vi "Bind RPC Register.vi"(11 "gRPCid server in":T1) -> (0 "error out":errorcluster, 1 "Register Internal UE":refnum<user-event>, 2 "Register gRPC UE":refnum<user-event>, 3 "gRPCid server out":T1)   [LabVIEW 2019, in "OOP Server.lvclass"]
uses:
  OOP Server.lvclass
  gRPC interface/Server API/typeDefs/gRPCId Cluster.ctl
  gRPC interface/Server API/typeDefs/grpcId.ctl
  typeDefs/gRPC Server Internal Message.ctl
  616620f9-6bbe-466a-af51-04bcc3596ea0.vi
  gRPC interface/gprc-lvsupport.lvlib
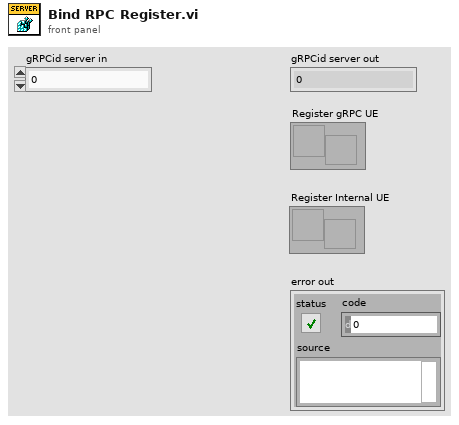
[diagram p1: front panel]
types:
  T1 = typedef "gprc-lvsupport.lvlib/grpcId.ctl" = u64
  T2 = typedef "OOP Server.lvclass/gRPC Server Internal Message.ctl" = cluster{"Command":string, "Data":variant}
  T3 = typedef "gprc-lvsupport.lvlib/gRPCId Cluster.ctl" = cluster{"gRPCid":T1}
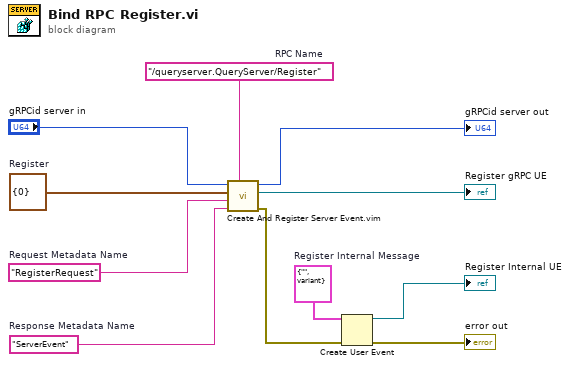
[diagram p0: block diagram]
diagram:
  w4 = T2 {"Command"="", "Data"=variant}  # Register Internal Message
  w7 = "ServerEvent"  # Response Metadata Name
  w10 = T3 {"gRPCid"=0}  # Register
  w8 = "RegisterRequest"  # Request Metadata Name
  w9 = "/queryserver.QueryServer/Register"  # RPC Name
  n1 = call "Create And Register Server Event.vim"("Method name"=w9, "Response Metadata Name"=w7, "Request Metadata Name"=w8, "event in"=w10, "gRPCid server in"="gRPCid server in") -> ("error out"=w2:errorcluster, "event"=→"Register gRPC UE":refnum<user-event>, "gRPCid server out"=→"gRPCid server out":T1)  [unwired: 4 in]
  n2 = Create User Event(user event datatype=w4, error in=w2) -> (user event=→"Register Internal UE":refnum<user-event>, error out=→"error out":errorcluster)
